vi "NIIE_Return MutationCode Folder.vi"() -> (3 "Base Path Mutation Code":path)   [LabVIEW 2021]
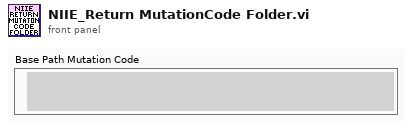
[diagram p1: front panel]
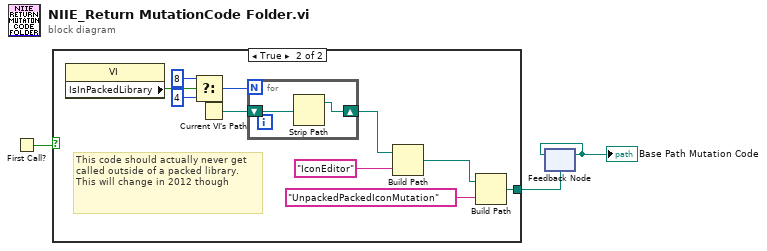
[diagram p0: block diagram]
diagram:
  n1 = First Call?() -> (First Call?: T/F=w1:bool)
  n2 = case shown="True" w1 {
    tunnel: [_ w5] -> w3
    frame False {
    }
    frame True {
      # "This code should actually never get\ncalled outside of a packed library. \nThis will change in 2012 though"
      n3 = property class="VI"() -> ("IsInPackedLibrary"=w9:bool)  [unwired: 2 in, 2 out]
      n4 = Select(t=8, s=w9, f=4) -> (s? t:f=w6:i32)
      n5 = Current VI's Path() -> (path=w4:path)
      n6 = for {
        N: w6 -> [_]
        shift-right: [w14] -> w13
        shift-left: w4 -> [w15]
        n7 = Strip Path(path=w15) -> (stripped path=w14:path)  [unwired: 1 out]
      }
      n8 = Build Path(base path=w13, name or relative path="IconEditor") -> (appended path=w10:path)
      n9 = Build Path(base path=w10, name or relative path="UnpackedPackedIconMutation") -> (appended path=w5:path)
    }
  }
  n10 = feedback #1(w3) -> (w2:path)
  "Base Path Mutation Code" <- w2
  n11 = feedback-in #1(w2) -> ()
